vi "Set ICommunicaters.vi"(10 "ICommunicaters":refnum<class "ICommunicate.lvclass">[](array[class]), 11 "Interactor in":refnum<class "Interactor.lvclass">) -> (3 "Interactor out":refnum<class "Interactor.lvclass">)   [LabVIEW 2024, in "Interactor.lvlib" / "Interactor.lvclass"]
uses:
  Interactor.lvclass
  Interactor.lvclass/Interactor.ctl
  HAL/Source/Interfaces/ICommunicate/ICommunicate.lvclass
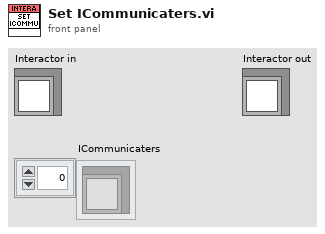
[diagram p1: front panel]
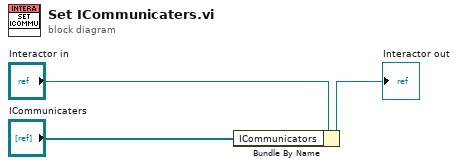
[diagram p0: block diagram]
diagram:
  n1 = Bundle By Name(cluster="Interactor in", "ICommunicators"="ICommunicaters") -> (→"Interactor out":refnum<class "Interactor.lvclass">)
